vi "outSensSel.vi"(8 "error in (no error)":errorcluster, 11 "Sensor Array":bool[](array[boolean])) -> (0 "error out":errorcluster, 3 "Sensor Selector":string)   [LabVIEW 2018]
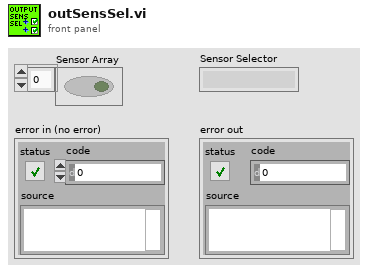
[diagram p1: front panel]
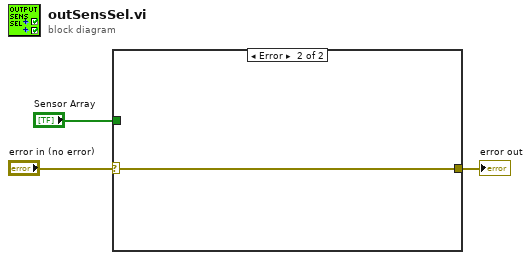
[diagram p0: block diagram]
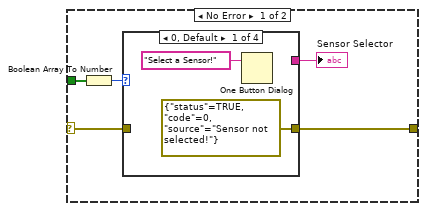
[diagram p2: hidden frame]
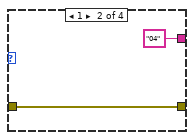
[diagram p3: hidden frame]
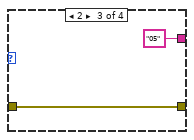
[diagram p4: hidden frame]
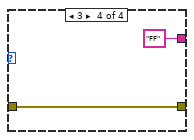
[diagram p5: hidden frame]
diagram:
  n1 = case shown="Error" "error in (no error)" {
    selector: "error in (no error)" -> [w4 w17]
    tunnel: [w7 w17] -> w3
    tunnel: "Sensor Array" -> [w5 _]
    frame No Error {
      n2 = Boolean Array To Number(Boolean array=w5) -> (number=w6:u32)
      n3 = case shown="0, Default" w6 {
        tunnel: w4 -> [_ w11 w13 w15]
        tunnel: [_ "04" "05" "FF"] -> w8
        tunnel: [errorcluster {"status"=TRUE, "code"=0, "source"="Sensor not selected!"} ("error constant") w11 w13 w15] -> w7
        frame 0, Default {
          n4 = One Button Dialog(message="Select a Sensor!") -> ()  [unwired: 1 in, 1 out]
        }
        frame 1 {
        }
        frame 2 {
        }
        frame 3 {
        }
      }
      "Sensor Selector" <- w8
    }
    frame Error {
    }
  }
  "error out" <- w3
